vi "Time_FGV.vi"(2 "에러 상수":errorcluster, 3 "상태":enum16{"초기화", "카운트", "정지"}(ring)) -> (0 "에러 상수 2":errorcluster caption="에러 상수", 1 "경과시간":dbl)   [LabVIEW 2020]
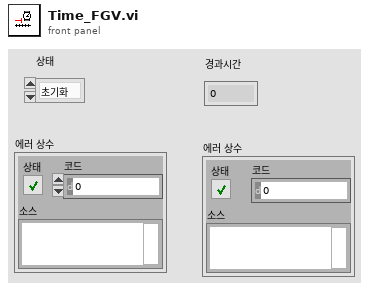
[diagram p1: front panel]
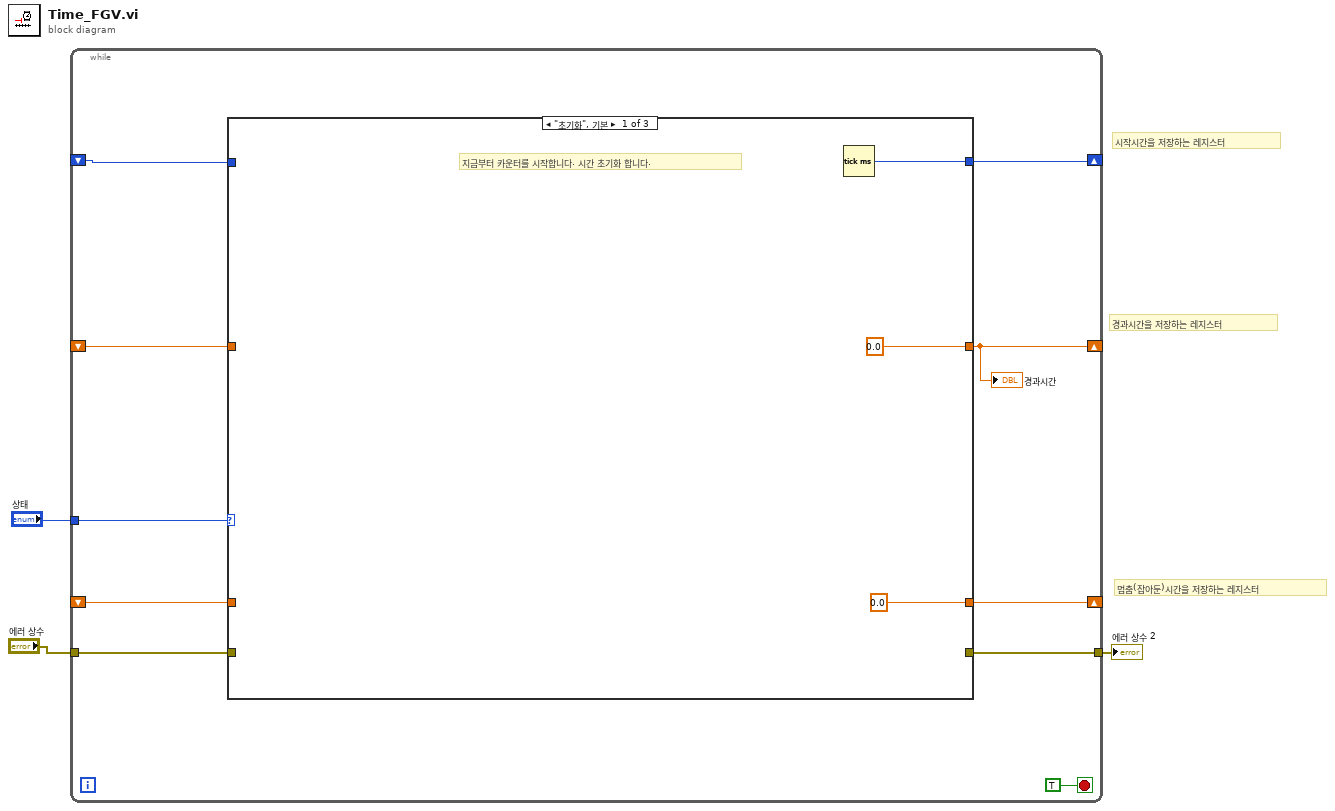
[diagram p0: block diagram]
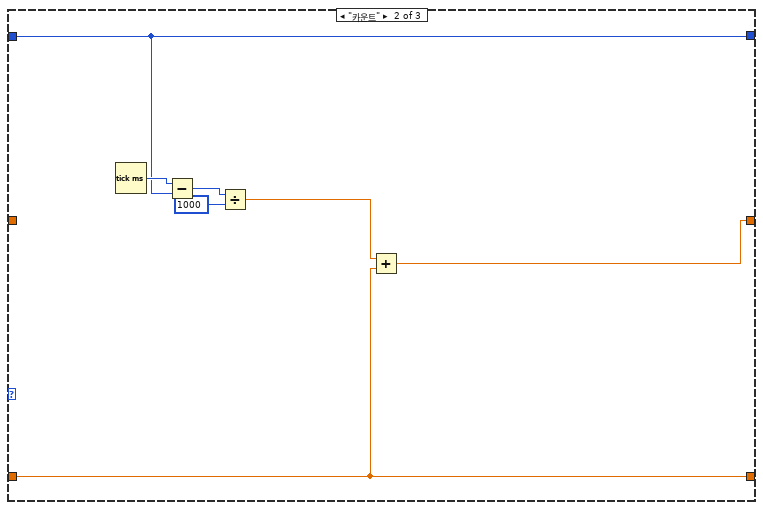
[diagram p2: hidden frame]
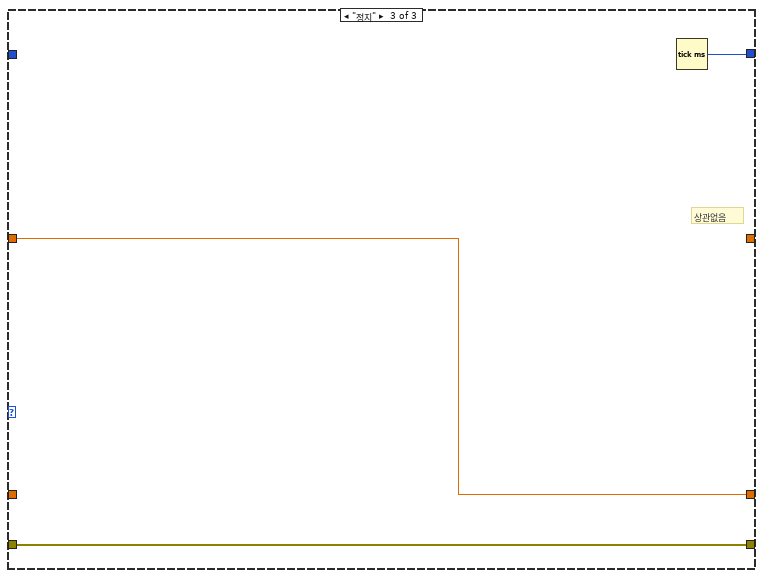
[diagram p3: hidden frame]
diagram:
  # "멈춤(잡아둔)시간을 저장하는 레지스터"
  # "경과시간을 저장하는 레지스터"
  # "시작시간을 저장하는 레지스터"
  n1 = while {
    shift-right: [w11] -> _
    shift-left: _ -> [w8]
    shift-right: [w10] -> _
    shift-left: _ -> [w6]
    shift-right: [w9] -> _
    shift-left: _ -> [w7]
    tunnel: "상태" -> [w12]
    tunnel: "에러 상수" -> [w5]
    tunnel: [w4] -> w1
    stop <- TRUE stop-if-true
    n2 = case shown="\"초기화\", 기본" w12 {
      tunnel: [w16 w20 w26] -> w11
      tunnel: [0.0 w18 _] -> w10
      tunnel: [0.0 w17 w25] -> w9
      tunnel: w8 -> [_ w20 _]
      tunnel: w7 -> [_ w17 _]
      tunnel: w6 -> [_ _ w25]
      tunnel: [_ _ w24] -> w4
      tunnel: w5 -> [_ _ w24]
      frame "초기화", Default {
        # "지금부터 카운터를 시작합니다. 시간 초기화 합니다."
        n3 = Tick Count (ms)() -> (millisecond timer value=w16:u32)
      }
      frame "카운트" {
        n4 = Tick Count (ms)() -> (millisecond timer value=w23:u32)
        n5 = Subtract(x=w23, y=w20) -> (x-y=w22:u32)
        n6 = Divide(x=w22, y=u32 1000) -> (x/y=w19:dbl)
        n7 = Add(x=w19, y=w17) -> (x+y=w18:dbl)
      }
      frame "정지" {
        # "상관없음"
        n8 = Tick Count (ms)() -> (millisecond timer value=w26:u32)
      }
    }
    "경과시간" <- w10
  }
  "에러 상수 2" <- w1
